vi "Scan.vi"(8 "error in (no error)":errorcluster, 11 "NI Galvo in":refnum<class "NI Galvo.lvclass">) -> (0 "error out":errorcluster, 3 "NI Galvo out":refnum<class "NI Galvo.lvclass">)   [LabVIEW 2014, in "NI Galvo.lvclass"]
uses:
  NI Galvo.lvclass
  NI Galvo.lvclass/NI Galvo.ctl
  Galvo.lvclass
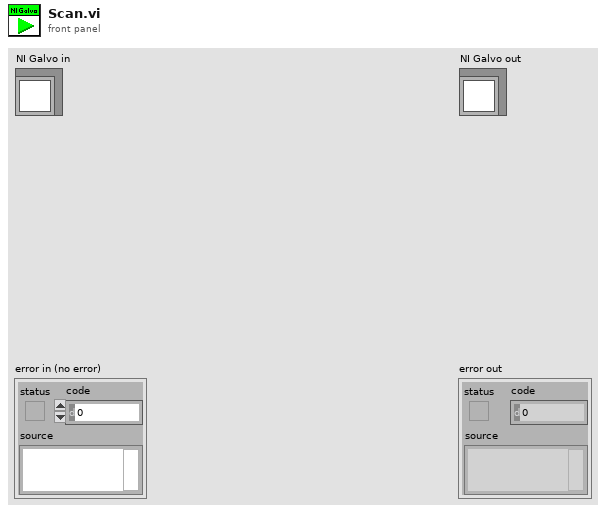
[diagram p1: front panel]
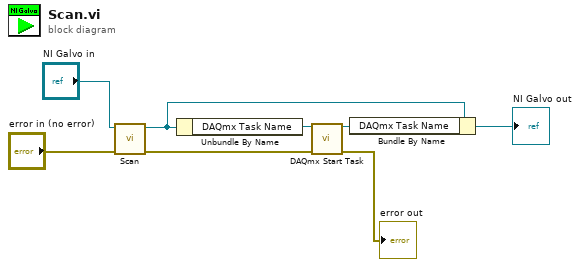
[diagram p0: block diagram]
diagram:
  n1 = call-parent "Scan.vi"("error in (no error)"="error in (no error)", "Galvo in"="NI Galvo in") -> ("error out"=w5:errorcluster, "Galvo out"=w4:refnum<class "NI Galvo.lvclass">)  [unwired: 8 in]
  n2 = Unbundle By Name(w4) -> ("DAQmx Task Name"=w6:refnum<k21>)
  n3 = call <vilib>:"DAQmx Start Task.vi"("task/channels in"=w6, "error in"=w5) -> ("task out"=w3:refnum<k21>, "error out"=→"error out":errorcluster)  [unwired: 12 in]
  n4 = Bundle By Name(cluster=w4, "DAQmx Task Name"=w3) -> (→"NI Galvo out":refnum<class "NI Galvo.lvclass">)
